vi "Test Password.vi"(8 "error in (no error)":errorcluster, 10 "String":string, 11 "TCP Network Connection in":refnum<k5>) -> (0 "error out":errorcluster, 1 "Authorized":T1, 2 "Password OK":bool)   [LabVIEW 2020]
doc: "Author: Scott Hannahs <sth@magnet.fsu.edu>\nCopyright 2018 Florida State University, All rights reserved."
uses:
  SCM4 Interlock LV20/RT SubVIs/RT System Auth Level.ctl
  TCP Functions/TCP Read Length and Value (STR).vi
  TCP Functions/TCP Write Length and Data (STR).vi
  TCP Functions/TCP Read Length and Value (U16).vi
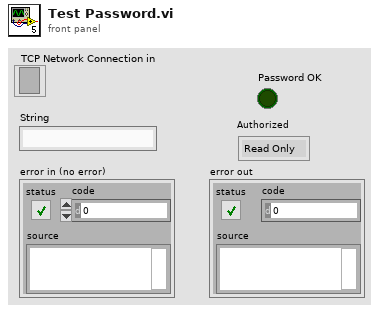
[diagram p1: front panel]
types:
  T1 = typedef "RT System Auth Level.ctl" = enum16{"Read Only", "User", "Operator", "Admin"}
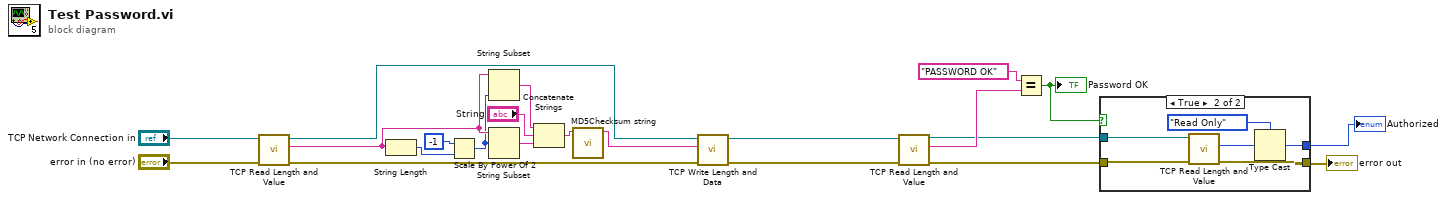
[diagram p0: block diagram]
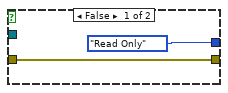
[diagram p2: hidden frame]
diagram:
  n1 = call-poly "TCP Read Length and Value.vi"("error in (no error)"="error in (no error)", "TCP Network Connection in"="TCP Network Connection in") -> ("error out"=w20:errorcluster, "Output"=w15:string, "TCP Network Connection out"=w12:refnum<k5>)  [unwired: 7 in]
  n2 = String Length(string=w15) -> (length=w7:i32)
  n3 = Scale By Power Of 2(n=i16 -1, x=w7) -> (x*2^n=w8:i32)
  n4 = String Subset(string=w15, length (rest)=w8) -> (substring=w17:string)  [unwired: 1 in]
  n5 = String Subset(string=w15, offset (0)=w8) -> (substring=w18:string)  [unwired: 1 in]
  n6 = Concatenate Strings(w17, "String", w18) -> (w19:string)
  n7 = call <vilib>:"MD5Checksum string.vi"("Message String"=w19) -> ("MD5 message-digest"=w10:string)  [unwired: 10 in]
  n8 = call-poly "TCP Write Length and Data.vi"("Error In"=w20, "Data"=w10, "connection ID"=w12) -> ("Error Out"=w21:errorcluster, "connection ID out"=w22:refnum<k5>)  [unwired: 7 in]
  n9 = call-poly "TCP Read Length and Value.vi"("error in (no error)"=w21, "TCP Network Connection in"=w22) -> ("error out"=w4:errorcluster, "Output"=w11:string, "TCP Network Connection out"=w2:refnum<k5>)  [unwired: 7 in]
  n10 = Equal?(x="PASSWORD OK" ("string"), y=w11) -> (x = y?=w5:bool)
  "Password OK" <- w5
  n11 = case shown="True" w5 {
    tunnel: w4 -> [w24 w29]
    tunnel: [w24 w28] -> w3
    tunnel: w2 -> [_ w30]
    tunnel: [RT_System_Auth_Level."Read Only" ("Authorized") w26] -> w1
    frame False {
    }
    frame True {
      n12 = call-poly "TCP Read Length and Value.vi"("error in (no error)"=w29, "TCP Network Connection in"=w30) -> ("error out"=w28:errorcluster, "Output"=w27:u16)  [unwired: 7 in, 1 out]
      n13 = Type Cast(type=RT_System_Auth_Level."Read Only" ("Authorized"), x=w27) -> (*(type *) &x=w26:T1)
    }
  }
  "error out" <- w3
  "Authorized" <- w1
